vi "TDMS Write Standard.vi"(8 "error in (no error)":errorcluster, 9 "Data":dbl[][](array[numeric]), 10 "Timestamps":timestamp[][](array[timestamp]), 11 "Path":path) -> (0 "error out":errorcluster, 2 "Time for Write (S)":dbl, 3 "Path Out":path)   [LabVIEW 2010]
doc: "Uses a common method of writing to file that will typically cause fragmentation. That is switching between writing timestamps and writing data channels."
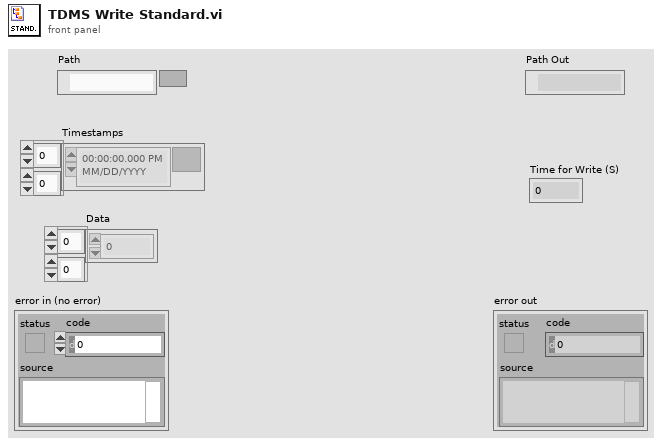
[diagram p1: front panel]
types:
  T1 = enum16{"open", "open or create", "create or replace", "create", "open (read-only)"}
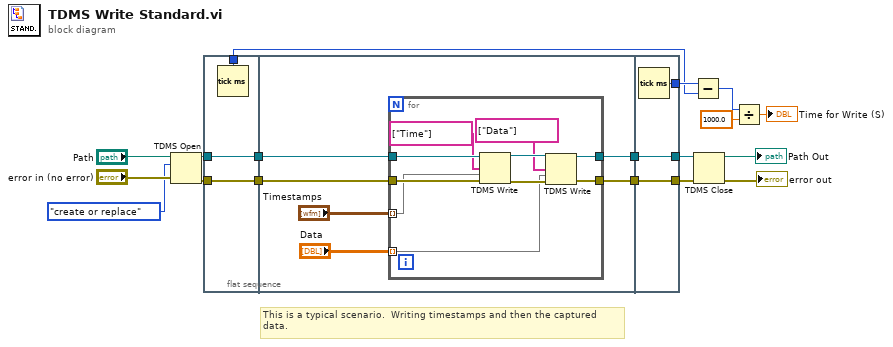
[diagram p0: block diagram]
diagram:
  # "This is a typical scenario.  Writing timestamps and then the captured\ndata."
  n1 = TDMS Open(8:"error in (no error)", 10:T1."create or replace" ("operation (0:open)"), 11:"Path") -> (0:w13:errorcluster, 3:w15:refnum<k34>)  [unwired: 3 in]
  n2 = flat-sequence {
    tunnel: [w21] -> w16
    tunnel: w15 -> [w21]
    tunnel: [w20] -> w14
    tunnel: w13 -> [w20]
    tunnel: [w19] -> w5
    tunnel: w16 -> [w25]
    tunnel: w14 -> [w24]
    tunnel: [w23] -> w8
    tunnel: [w22] -> w7
    tunnel: [w39] -> w11
    tunnel: [w40] -> w12
    tunnel: w8 -> [w40]
    tunnel: w7 -> [w39]
    tunnel: [w38] -> w6
    frame #0 {
      n3 = Tick Count (ms)() -> (millisecond timer value=w19:u32)
    }
    frame #1 {
      n4 = for {
        tunnel: "Timestamps" -> [w31] mode=indexing
        tunnel: "Data" -> [w30] mode=indexing
        tunnel: w25 -> [w37]
        tunnel: w24 -> [w36]
        tunnel: [w29] -> w23
        tunnel: [w28] -> w22
        n5 = TDMS Write(0:w37, 7:string[] ["Time"] ("channel name(s) in (Untitled)"), 9:w31, 11:w36) -> (4:w35:refnum<k34>, 15:w34:errorcluster)  [unwired: 2 in, 2 out]
        n6 = TDMS Write(0:w35, 7:string[] ["Data"] ("channel name(s) in (Untitled)"), 9:w30, 11:w34) -> (4:w29:refnum<k34>, 15:w28:errorcluster)  [unwired: 2 in, 2 out]
      }
    }
    frame #2 {
      n7 = Tick Count (ms)() -> (millisecond timer value=w38:u32)
    }
  }
  n8 = Subtract(x=w6, y=w5) -> (x-y=w4:u32)
  n9 = TDMS Close(8:w11, 11:w12) -> (0:→"error out":errorcluster, 3:→"Path Out":path)
  n10 = Divide(x=w4, y=1000.0) -> (x/y=→"Time for Write (S)":dbl)
